vi "Get Library Info.vi"(8 "error in (no error)":errorcluster) -> (0 "error out":errorcluster, 1 "License":string, 2 "Copyright":string, 3 "Version String":string, 5 "Name":string)   [LabVIEW 2009, in "Caraya.lvlib"]
uses:
  Caraya.lvlib
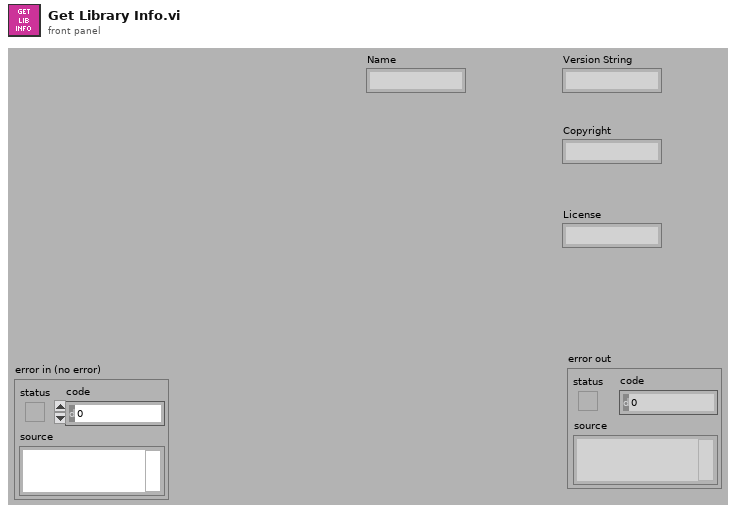
[diagram p1: front panel]
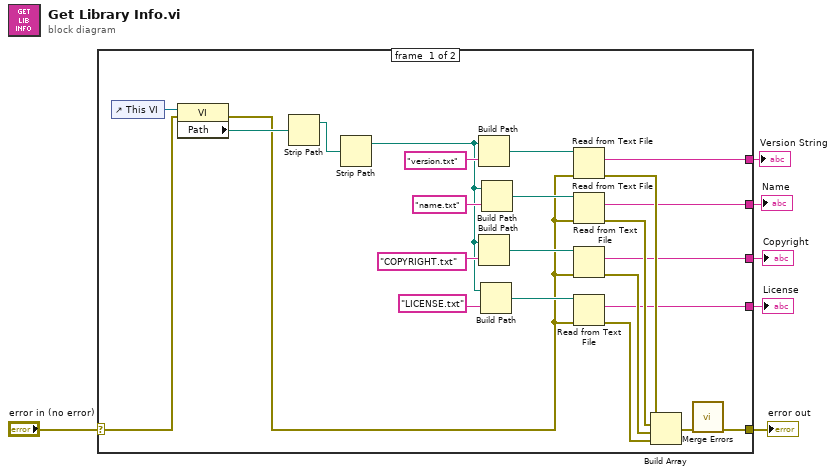
[diagram p0: block diagram]
diagram:
  n1 = case shown="No Error" "error in (no error)" {
    selector: "error in (no error)" -> [w29 w31]
    tunnel: [w10 w31] -> w5
    tunnel: [w26 _] -> w4
    tunnel: [w9 _] -> w3
    tunnel: [w8 _] -> w2
    tunnel: [w7 _] -> w1
    frame #0 {
      n2 = control-ref of="This VI"() -> (w30:refnum<vi>)
      n3 = property class="VI"(reference=w30, error in=w29) -> (error out=w12:errorcluster, "Path"=w25:path)  [unwired: 1 out]
      n4 = Strip Path(path=w25) -> (stripped path=w24:path)  [unwired: 1 out]
      n5 = Strip Path(path=w24) -> (stripped path=w20:path)  [unwired: 1 out]
      n6 = Build Path(base path=w20, name or relative path="version.txt") -> (appended path=w27:path)
      n7 = Build Path(base path=w20, name or relative path="COPYRIGHT.txt") -> (appended path=w18:path)
      n8 = Build Path(base path=w20, name or relative path="LICENSE.txt") -> (appended path=w17:path)
      n9 = Build Path(base path=w20, name or relative path="name.txt") -> (appended path=w19:path)
      n10 = Read from Text File(file (use dialog)=w27, error in=w12) -> (text=w26:string, error out=w16:errorcluster)  [unwired: 2 in, 2 out]
      n11 = Read from Text File(file (use dialog)=w19, error in=w12) -> (text=w9:string, error out=w15:errorcluster)  [unwired: 2 in, 2 out]
      n12 = Read from Text File(file (use dialog)=w18, error in=w12) -> (text=w8:string, error out=w14:errorcluster)  [unwired: 2 in, 2 out]
      n13 = Read from Text File(file (use dialog)=w17, error in=w12) -> (text=w7:string, error out=w13:errorcluster)  [unwired: 2 in, 2 out]
      n14 = Build Array(w16, w15, w14, w13) -> (w11:errorcluster[])
      n15 = call <vilib>:"Merge Errors.vi"("error array in"=w11) -> ("error out"=w10:errorcluster)  [unwired: 6 in]
    }
    frame #1 {
    }
  }
  "error out" <- w5
  "Version String" <- w4
  "Name" <- w3
  "Copyright" <- w2
  "License" <- w1
